vi "ExtractGraphs.vi"(0 "Spectra Out":T1[](array[typedef]) {"Settings"."Time" format="%<%H:%M\n%d/%m/%y>T"}) -> (1 "Plot Labels":string[](array[string]), 2 "Mag":cluster{i32, dbl, "data":dbl[]}[](graph), 3 "Plot type":enum16{"Linear", "log"}(ring), 4 "FileNames":string[](array[string]))   [LabVIEW 2014]
uses:
  <userlib>/CurtinCode/DataControl.ctl
  <userlib>/CurtinCode/SettingsControl.ctl
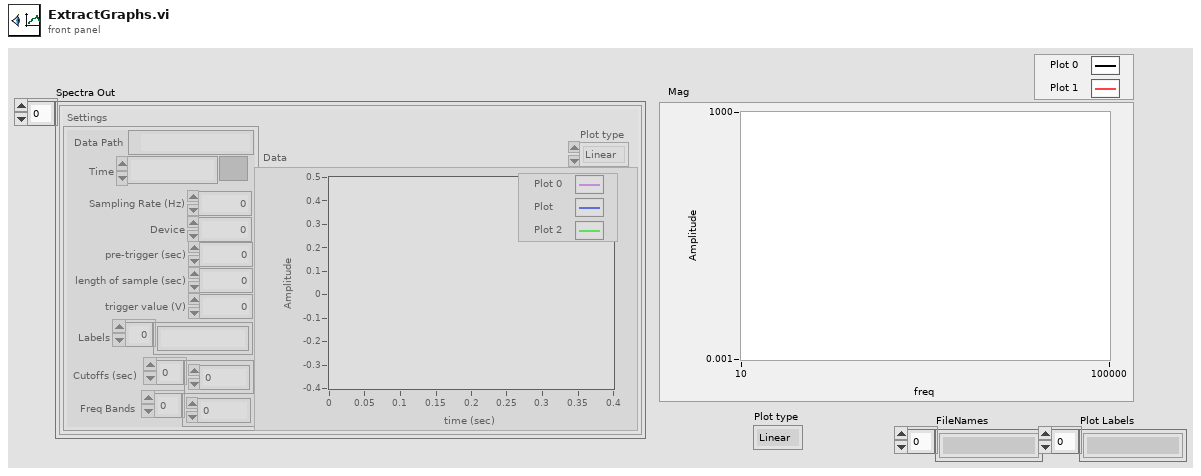
[diagram p1: front panel]
types:
  T1 = typedef "DataControl.ctl" = cluster{"Settings":T2, "Data":cluster{i32, dbl, "data":dbl[]}[], "Plot type":enum16{"Linear", "log"}}
  T2 = typedef "SettingsControl.ctl" = cluster{"Data Path":path, "Time":timestamp, "Sampling Rate (Hz)":u16, "Device":u16, "pre-trigger (sec)":dbl, "length of sample (sec)":dbl, "trigger value (V)":dbl, "Labels":string[], "Cutoffs (sec)":dbl[], "Freq Bands":dbl[]}
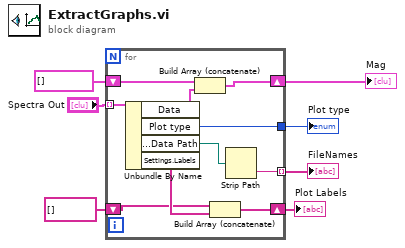
[diagram p0: block diagram]
diagram:
  n1 = for {
    tunnel: "Spectra Out" -> [w17] mode=indexing
    shift-right: [w16] -> w6
    shift-left: cluster{i32, dbl, "data":dbl[]}[] [] -> [w14]
    tunnel: [w13] -> w4
    tunnel: [w11] -> w3 mode=indexing
    shift-right: [w9] -> w1
    shift-left: string[] [] -> [w8]
    n2 = Unbundle By Name(w17) -> ("Data"=w15:cluster{i32, dbl, "data":dbl[]}[], "Plot type"=w13:enum16{"Linear", "log"}, "Settings.Data Path"=w12:path, "Settings.Labels"=w10:string[])
    n3 = Build Array (concatenate)(w14, w15) -> (w16:cluster{i32, dbl, "data":dbl[]}[])
    n4 = Build Array (concatenate)(w8, w10) -> (w9:string[])
    n5 = Strip Path(path=w12) -> (name=w11:string)  [unwired: 1 out]
  }
  "Mag" <- w6
  "Plot type" <- w4
  "FileNames" <- w3
  "Plot Labels" <- w1
